vi "LVClass_WavefrontCorrectorSet ReadFile WavefrontCorrectorSetup.vi"(0 "WavefrontCorrectorSet in":refnum<class "WavefrontCorrectorSet.lvclass">, 11 "error in (no error)":errorcluster) -> (4 "WavefrontCorrectorSet out":refnum<class "WavefrontCorrectorSet.lvclass">, 15 "error out":errorcluster)   [LabVIEW 2020, in "WavefrontCorrectorSet.lvclass"]
uses:
  WavefrontCorrectorSet.lvclass
  WavefrontCorrectorSet.lvclass/WavefrontCorrectorSet.ctl
  CameraParametersSetup.ctl
  CameraParameters_Type.ctl
  File Exists - Scalar__ogtk.vi
  <vilib>/Utility/xml.llb/Read From XML File(string).vi
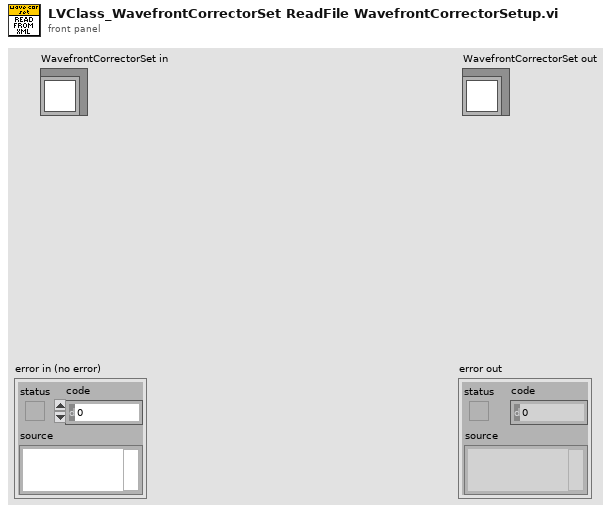
[diagram p1: front panel]
types:
  T1 = typedef "CameraParametersSetup.ctl" = cluster{"Name":string, "Type":T2, "Value":dbl, "BooleanValue":bool, "StringValue":string, "ConnectionParameter":bool}
  T2 = typedef "CameraParameters_Type.ctl" = enum16{"Integer", "Real", "String", "Boolean"}
  T3 = typedef "Wavefront Corrector states - ONE.ctl" = cluster{"Max":sgl, "Min":sgl, "Validity":enum16{"valid", "fixed", "invalid"}, "Fixed_Position":sgl}
  T4 = typedef "Wavefront Corrector states.ctl" = cluster{"Sleep after command apply_ms":i32, "Wavefront Corrector State":T3[], "WavefrontCorrectorOffsetState":sgl[]}
  T5 = typedef "ParameterID.ctl" = cluster{"Name":string, "ConnectionParameter?":bool, "Type":T2, "Authorization":T6, "OnFlyAuthorization":T7, "StringValue":string, "Value":dbl, "Min":dbl, "Max":dbl, "BooleanValue":bool, "StringParameterList":string[]}
  T6 = typedef "CameraParameters_Authorization.ctl" = enum16{"Disable", "Gettable", "Settable - Gettable"}
  T7 = typedef "CameraParameters_OnFlyAuthorization.ctl" = enum16{"None", "Gettable", "Settable", "Settable - Gettable"}
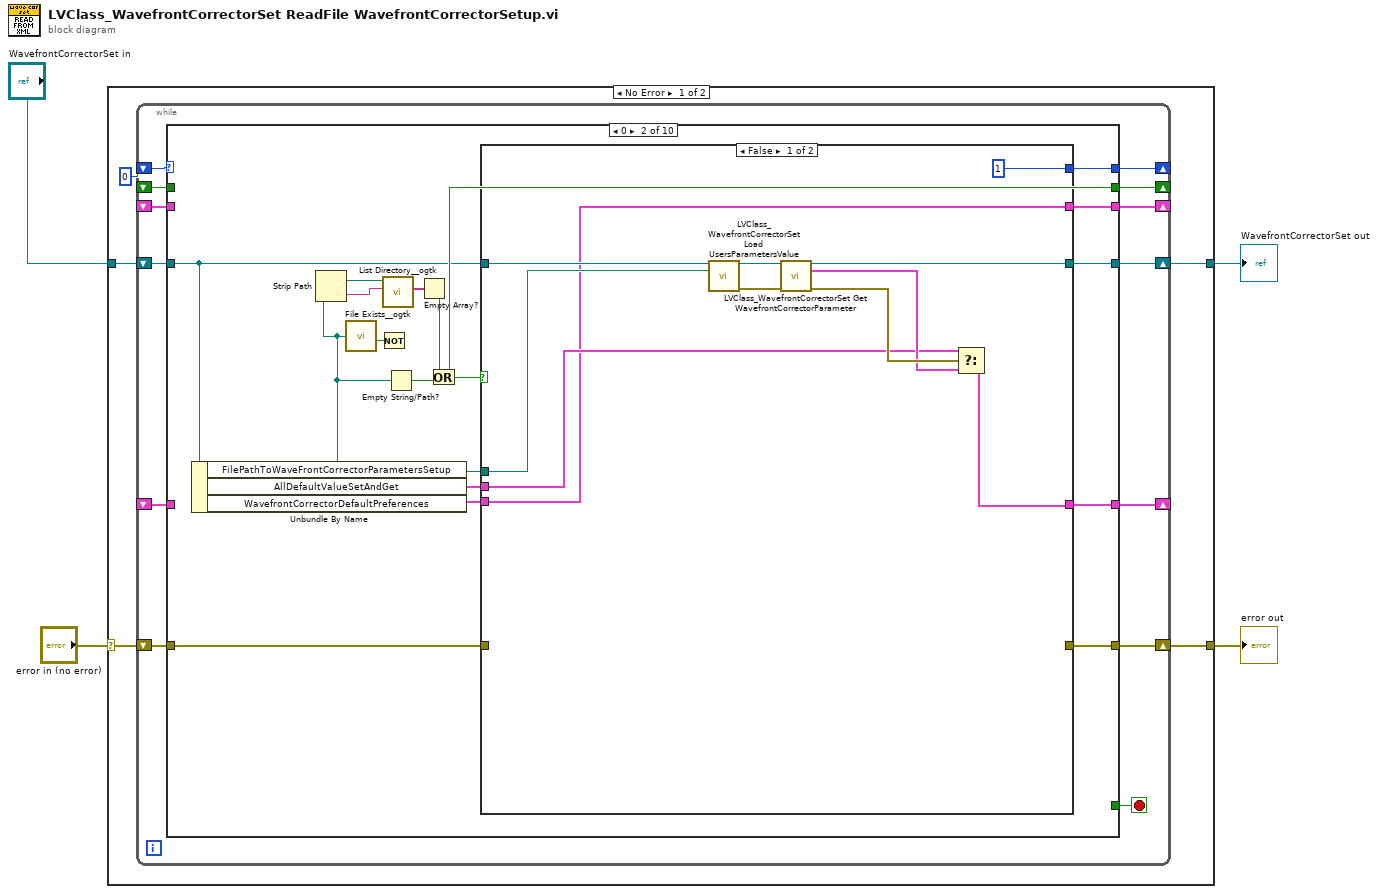
[diagram p0: block diagram]
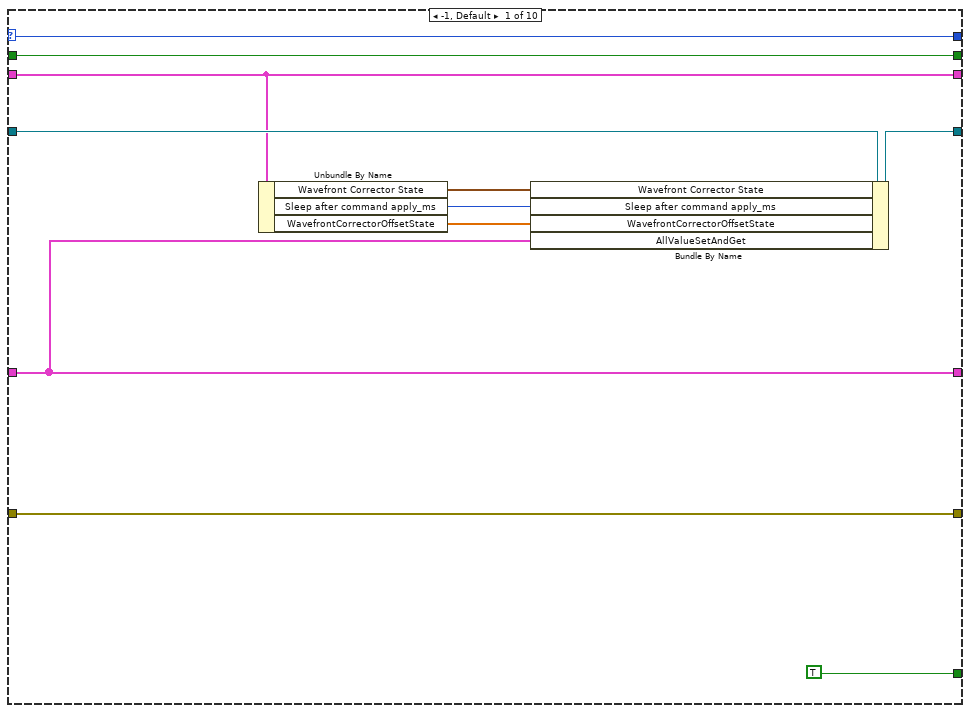
[diagram p2: hidden frame]
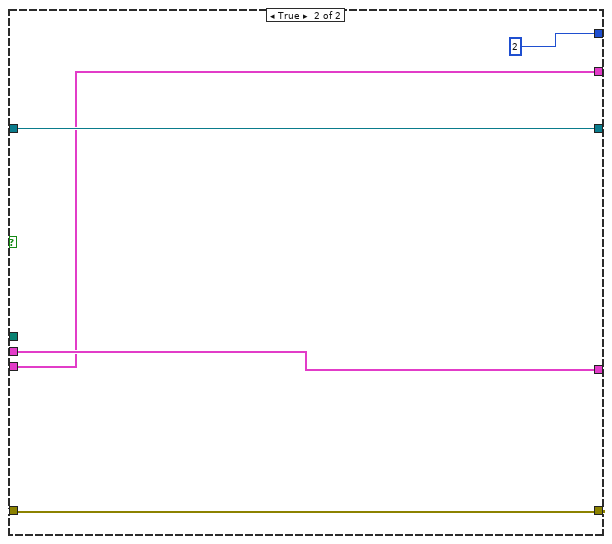
[diagram p3: hidden frame]
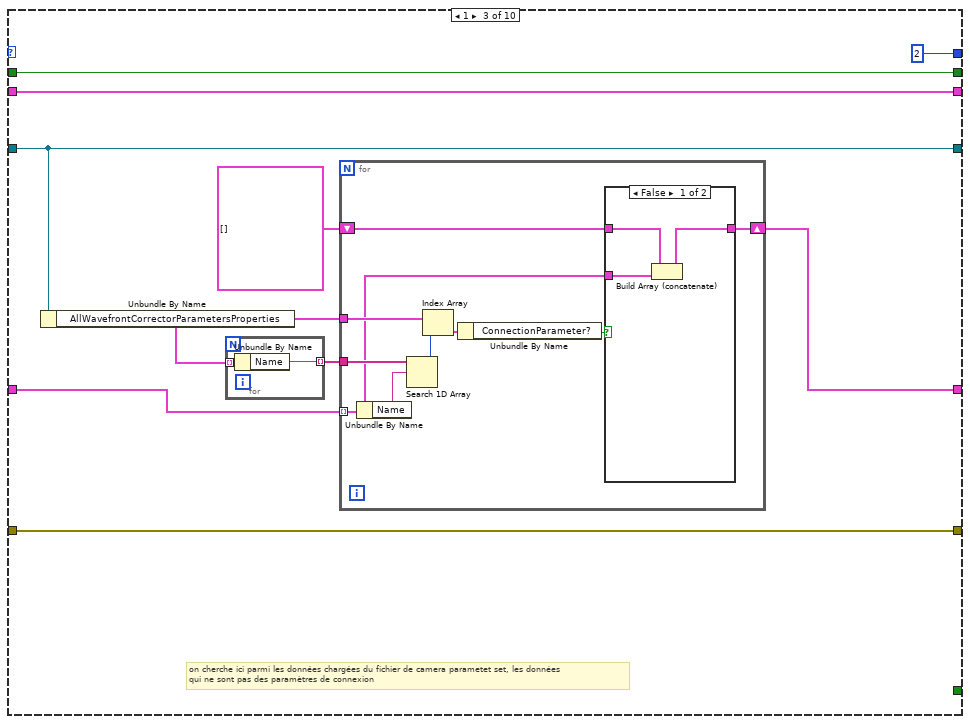
[diagram p4: hidden frame]
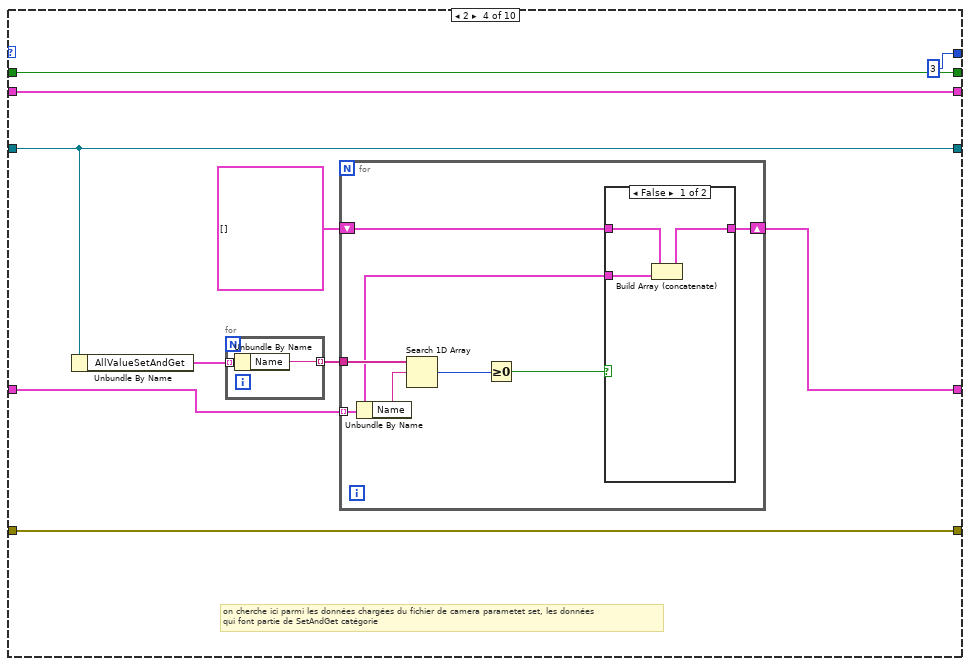
[diagram p6: hidden frame]
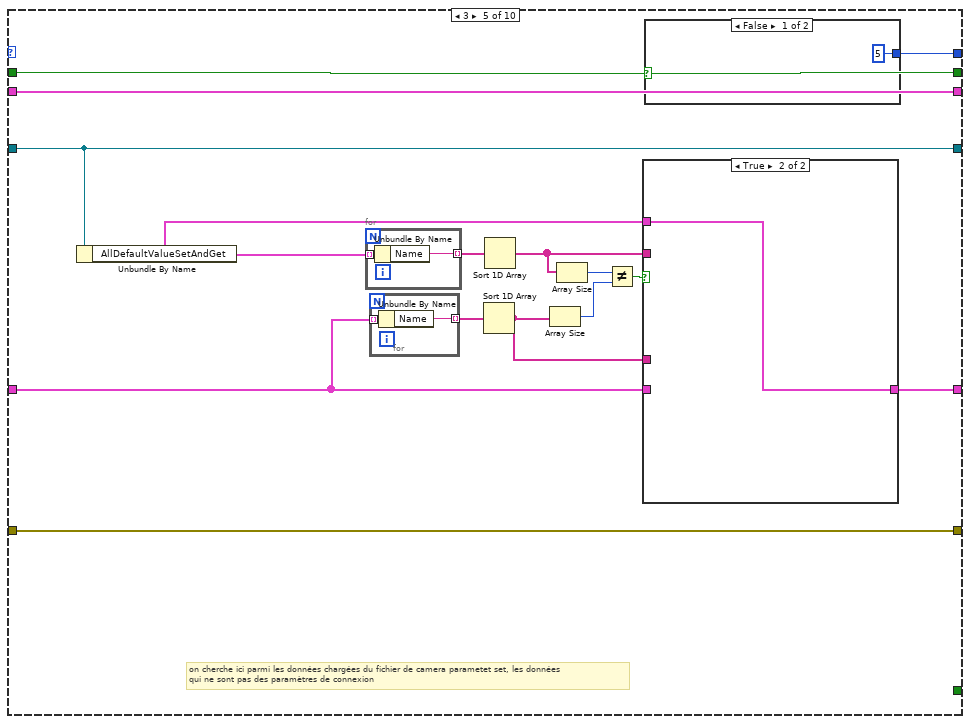
[diagram p8: hidden frame]
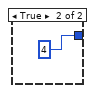
[diagram p9: hidden frame]
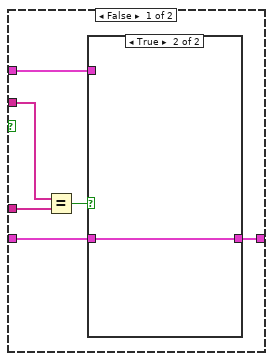
[diagram p10: hidden frame]
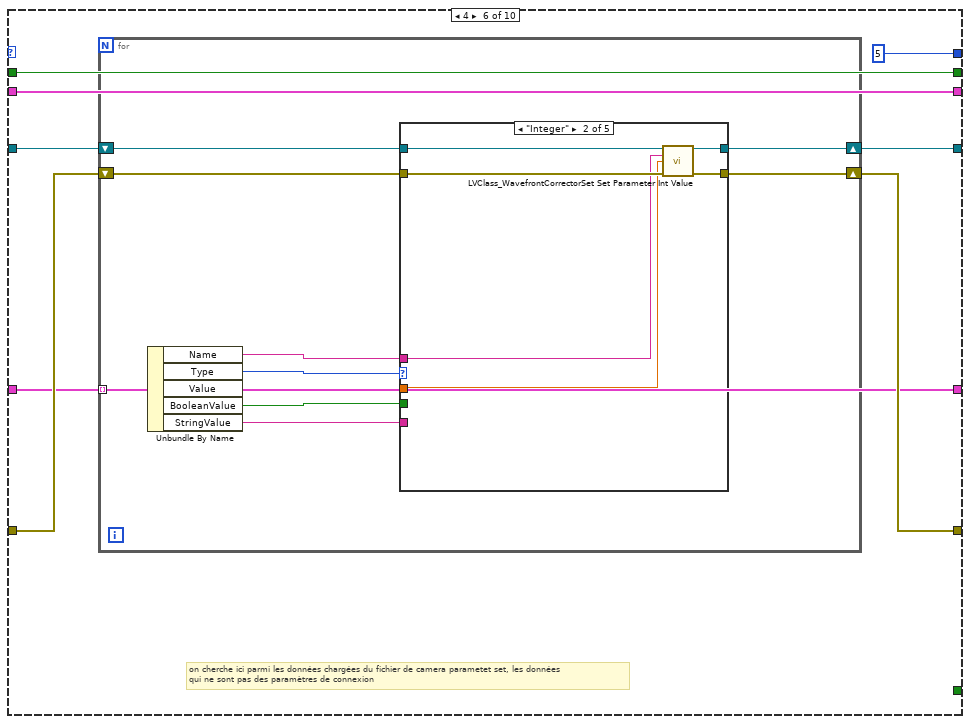
[diagram p12: hidden frame]
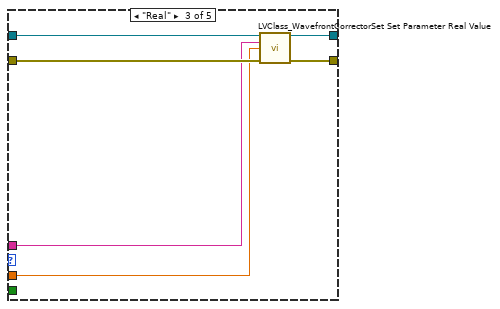
[diagram p14: hidden frame]
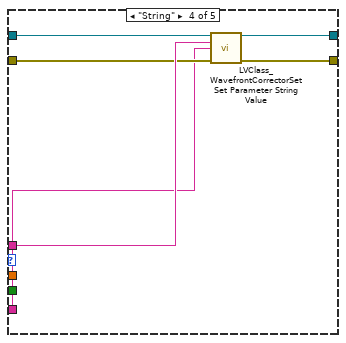
[diagram p15: hidden frame]
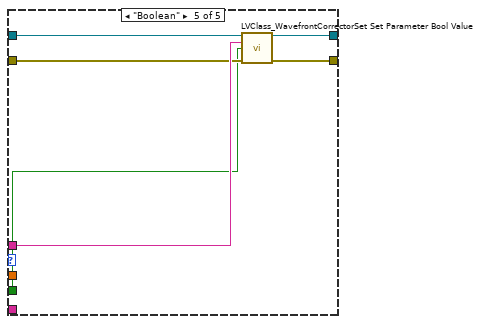
[diagram p16: hidden frame]
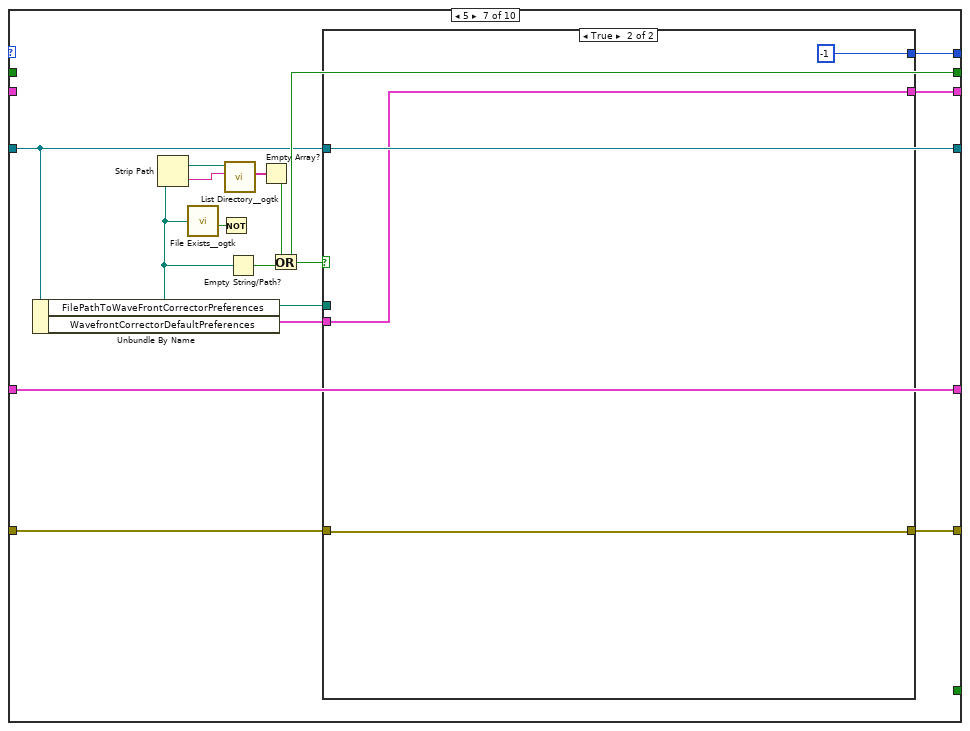
[diagram p17: hidden frame]
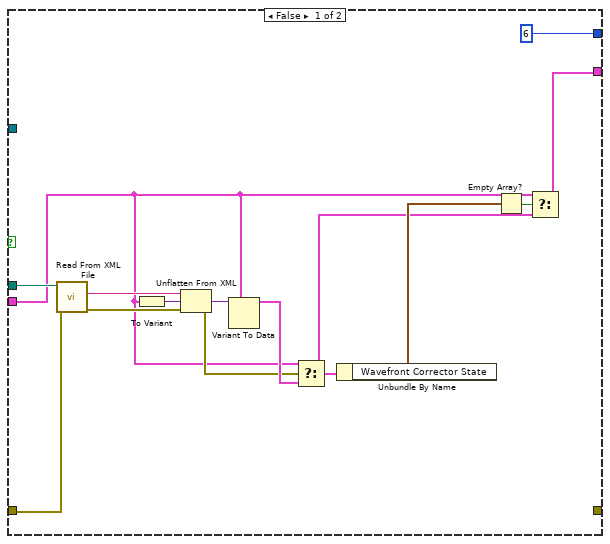
[diagram p18: hidden frame]
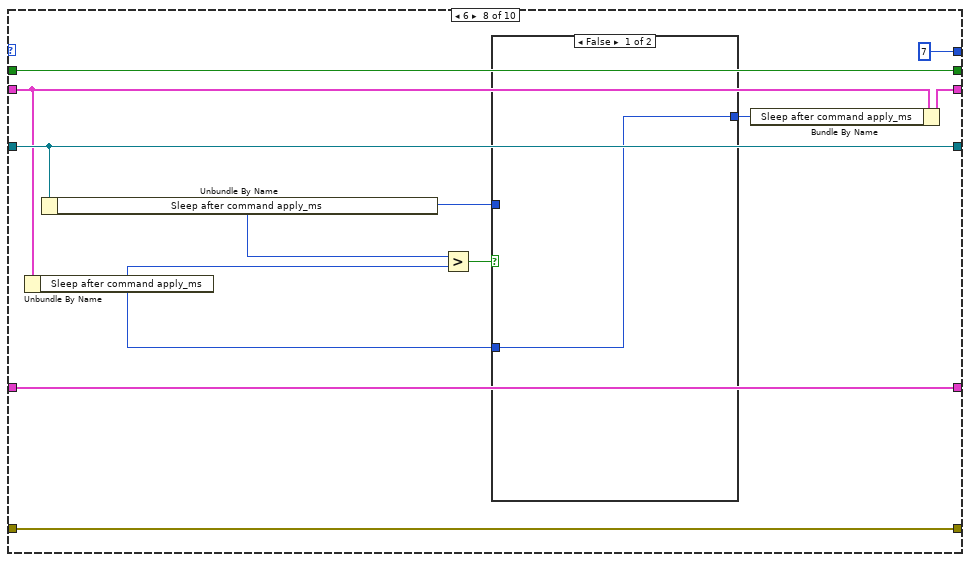
[diagram p19: hidden frame]
diagram:
  n1 = case shown="No Error" "error in (no error)" {
    selector: "error in (no error)" -> [w8 w265]
    tunnel: [w9 w265] -> w3
    tunnel: "WavefrontCorrectorSet in" -> [w6 w264]
    tunnel: [w5 w264] -> w1
    frame No Error {
      n2 = while {
        shift-right: [w20] -> _
        shift-left: _ -> [w16]
        shift-right: [w14] -> _
        shift-left: 0 -> [w18]
        shift-right: [w15] -> w5
        shift-left: w6 -> [w19]
        shift-right: [w22] -> w9
        shift-left: w8 -> [w21]
        shift-right: [w10] -> _
        shift-left: _ -> [w13]
        shift-right: [w11] -> _
        shift-left: _ -> [w12]
        stop <- w17 stop-if-true
        n3 = case shown="0" w18 {
          selector: w18 -> [w31 _ _ _ _ _ _ _ _ _]
          tunnel: [w32 w50 w75 w100 w124 w146 w203 w229 w241 w256] -> w22
          tunnel: w21 -> [w32 w49 w75 w100 w124 w147 w202 w229 w241 w256]
          tunnel: [w26 w48 w68 w93 w116 w150 w201 w221 w234 w249] -> w20
          tunnel: w19 -> [w30 w34 w71 w96 w129 w149 w189 w230 w245 w260]
          tunnel: [TRUE _ _ _ _ _ _ _ _ _] -> w17
          tunnel: w16 -> [w26 _ w68 w93 w116 w150 _ w222 w235 w250]
          tunnel: [w29 w37 w71 w96 w129 w148 w189 w230 w245 w260] -> w15
          tunnel: [w31 w46 2 3 w118 5 w200 7 8 -1] -> w14
          tunnel: [w27 w35 w69 w94 w119 w145 w190 w228 w238 w253] -> w10
          tunnel: w13 -> [w27 _ w70 w95 w117 w145 w190 w228 w238 w253]
          tunnel: w12 -> [w28 _ w67 w92 w115 w151 _ w224 w237 w252]
          tunnel: [w28 w36 w67 w92 w115 w151 w191 w224 w237 w252] -> w11
          frame -1, Default {
            n4 = Unbundle By Name(w26) -> ("Wavefront Corrector State"=w23:T3[], "Sleep after command apply_ms"=w24:i32, "WavefrontCorrectorOffsetState"=w25:sgl[])
            n5 = Bundle By Name(cluster=w30, "Wavefront Corrector State"=w23, "Sleep after command apply_ms"=w24, "WavefrontCorrectorOffsetState"=w25, "AllValueSetAndGet"=w27) -> (w29:refnum<class "WavefrontCorrectorSet.lvclass">)
          }
          frame 0 {
            n6 = Unbundle By Name(w34) -> ("FilePathToWaveFrontCorrectorParametersSetup"=w38:path, "AllDefaultValueSetAndGet"=w47:T1[], "WavefrontCorrectorDefaultPreferences"=w45:T4)
            n7 = Strip Path(path=w38) -> (stripped path=w41:path, name=w40:string)
            n8 = call-poly "File Exists__ogtk.vi"("file path"=w38) -> ("exists"=w39:bool)  [unwired: 6 in, 1 out]
            n9 = Not(x=w39) -> ()  [unwired: 1 out]
            n10 = call "List Directory__ogtk.vi"("pattern"=w40, "directory path"=w41) -> ("file names"=w42:string[])  [unwired: 2 in, 3 out]
            n11 = Empty String/Path?(string/path=w38) -> (empty?=w44:bool)
            n12 = Empty Array?(array=w42) -> (empty?=w43:bool)
            n13 = Or(x=w43, y=w44) -> (x .or. y?=w36:bool)
            n14 = case shown="False" w36 {
              tunnel: w38 -> [w58 _]
              tunnel: [_ w66] -> w50
              tunnel: w49 -> [_ w66]
              tunnel: [w51 w62] -> w48
              tunnel: w47 -> [w53 w63]
              tunnel: [1 2] -> w46
              tunnel: w45 -> [w51 w62]
              tunnel: w34 -> [w59 w64]
              tunnel: [w56 w64] -> w37
              tunnel: [w52 w63] -> w35
              frame False {
                n15 = call "LVClass_WavefrontCorrectorSet Load UsersParametersValue.vi"("WavefrontCorrectorSet in"=w59, "ParametersValue file path"=w58) -> ("WavefrontCorrectorSet out"=w57:refnum<class "WavefrontCorrectorSet.lvclass">, "error out"=w60:errorcluster)  [unwired: 12 in]
                n16 = call "LVClass_WavefrontCorrectorSet Get WavefrontCorrectorParameter.vi"("WavefrontCorrectorSet in"=w57, "error in (no error)"=w60) -> ("WavefrontCorrectorSet out"=w56:refnum<class "WavefrontCorrectorSet.lvclass">, "AllCurrentValueSetAndGet"=w54:T1[], "error out"=w55:errorcluster)  [unwired: 10 in, 1 out]
                n17 = Select(t=w53, s=w55, f=w54) -> (s? t:f=w52:T1[])
              }
              frame True {
              }
            }
          }
          frame 1 {
            # "on cherche ici parmi les données chargées du fichier de camera parametet set, les données \nqui ne sont pas des paramètres de connexion"
            n18 = Unbundle By Name(w71) -> ("AllWavefrontCorrectorParametersProperties"=w73:T5[])
            n19 = for {
              tunnel: w73 -> [w78] mode=indexing
              tunnel: [w77] -> w72 mode=indexing
              n20 = Unbundle By Name(w78) -> ("Name"=w77:string)
            }
            n21 = for {
              tunnel: w72 -> [w87]
              tunnel: w70 -> [w81] mode=indexing
              tunnel: w73 -> [w85]
              shift-right: [w82] -> w69
              shift-left: T1[] [] -> [w83]
              n22 = Unbundle By Name(w81) -> ("Name"=w86:string)
              n23 = Search 1D Array(1D array=w87, element=w86) -> (index of element=w84:i32)  [unwired: 1 in]
              n24 = Index Array(array=w85, index=w84) -> (element=w80:T5)
              n25 = Unbundle By Name(w80) -> ("ConnectionParameter?"=w79:bool)
              n26 = case shown="False" w79 {
                tunnel: w83 -> [w90 w91]
                tunnel: [w89 w91] -> w82
                tunnel: w81 -> [w88 _]
                frame False {
                  n27 = Build Array (concatenate)(w90, w88) -> (w89:T1[])
                }
                frame True {
                }
              }
            }
          }
          frame 2 {
            # "on cherche ici parmi les données chargées du fichier de camera parametet set, les données \nqui font partie de SetAndGet catégorie"
            n28 = Unbundle By Name(w96) -> ("AllValueSetAndGet"=w98:T1[])
            n29 = for {
              tunnel: w98 -> [w103] mode=indexing
              tunnel: [w102] -> w97 mode=indexing
              n30 = Unbundle By Name(w103) -> ("Name"=w102:string)
            }
            n31 = for {
              tunnel: w97 -> [w110]
              tunnel: w95 -> [w106] mode=indexing
              shift-right: [w107] -> w94
              shift-left: T1[] [] -> [w108]
              n32 = Unbundle By Name(w106) -> ("Name"=w109:string)
              n33 = Search 1D Array(1D array=w110, element=w109) -> (index of element=w105:i32)  [unwired: 1 in]
              n34 = Greater Or Equal To 0?(x=w105) -> (x >= 0?=w104:bool)
              n35 = case shown="False" w104 {
                tunnel: w108 -> [w113 w114]
                tunnel: [w112 w114] -> w107
                tunnel: w106 -> [w111 _]
                frame False {
                  n36 = Build Array (concatenate)(w113, w111) -> (w112:T1[])
                }
                frame True {
                }
              }
            }
          }
          frame 3 {
            # "on cherche ici parmi les données chargées du fichier de camera parametet set, les données \nqui ne sont pas des paramètres de connexion"
            n37 = Unbundle By Name(w129) -> ("AllDefaultValueSetAndGet"=w125:T1[])
            n38 = for {
              tunnel: w125 -> [w142] mode=indexing
              tunnel: [w141] -> w122 mode=indexing
              n39 = Unbundle By Name(w142) -> ("Name"=w141:string)
            }
            n40 = for {
              tunnel: w117 -> [w144] mode=indexing
              tunnel: [w143] -> w120 mode=indexing
              n41 = Unbundle By Name(w144) -> ("Name"=w143:string)
            }
            n42 = Sort 1D Array(array=w120) -> (sorted array=w121:string[])
            n43 = Sort 1D Array(array=w122) -> (sorted array=w123:string[])
            n44 = Array Size(array=w121) -> (size(s)=w127:i32)
            n45 = Array Size(array=w123) -> (size(s)=w128:i32)
            n46 = Not Equal?(x=w128, y=w127) -> (x != y?=w126:bool)
            n47 = case shown="True" w126 {
              tunnel: w125 -> [w132 w140]
              tunnel: [w134 w140] -> w119
              tunnel: w123 -> [w137 _]
              tunnel: w121 -> [w136 _]
              tunnel: w117 -> [w133 _]
              frame False {
                n48 = Equal?(x=w137, y=w136) -> (x = y?=w135:bool)
                n49 = case shown="True" w135 {
                  tunnel: [w138 w139] -> w134
                  tunnel: w133 -> [_ w139]
                  tunnel: w132 -> [w138 _]
                  frame False {
                  }
                  frame True {
                  }
                }
              }
              frame True {
              }
            }
            n50 = case shown="False" w115 {
              tunnel: [5 4] -> w118
              frame False {
              }
              frame True {
              }
            }
          }
          frame 4 {
            # "on cherche ici parmi les données chargées du fichier de camera parametet set, les données \nqui ne sont pas des paramètres de connexion"
            n51 = for {
              tunnel: w145 -> [w155] mode=indexing
              shift-right: [w156] -> w148
              shift-left: w149 -> [w157]
              shift-right: [w153] -> w146
              shift-left: w147 -> [w154]
              n52 = Unbundle By Name(w155) -> ("Name"=w158:string, "Type"=w162:T2, "Value"=w159:dbl, "BooleanValue"=w161:bool, "StringValue"=w160:string)
              n53 = case shown="\"Integer\"" w162 {
                tunnel: w158 -> [_ w165 w172 w181 w187]
                tunnel: w157 -> [w164 w170 w176 w182 w188]
                tunnel: [w164 w168 w174 w179 w185] -> w156
                tunnel: [w163 w167 w173 w178 w184] -> w153
                tunnel: w154 -> [w163 w169 w175 w180 w186]
                tunnel: w159 -> [_ w166 w171 _ _]
                tunnel: w161 -> [_ _ _ _ w183]
                tunnel: w160 -> [_ _ _ w177 _]
                frame Default {
                }
                frame "Integer" {
                  n54 = call "LVClass_WavefrontCorrectorSet Set Parameter Int Value.vi"("WavefrontCorrectorSet in"=w170, "parameter_name"=w165, "Value"=w166, "error in (no error)"=w169) -> ("WavefrontCorrectorSet out"=w168:refnum<class "WavefrontCorrectorSet.lvclass">, "error out"=w167:errorcluster)  [unwired: 10 in]
                }
                frame "Real" {
                  n55 = call "LVClass_WavefrontCorrectorSet Set Parameter Real Value.vi"("WavefrontCorrectorSet in"=w176, "parameter_name"=w172, "Value"=w171, "error in (no error)"=w175) -> ("WavefrontCorrectorSet out"=w174:refnum<class "WavefrontCorrectorSet.lvclass">, "error out"=w173:errorcluster)  [unwired: 10 in]
                }
                frame "String" {
                  n56 = call "LVClass_WavefrontCorrectorSet Set Parameter String Value.vi"("WavefrontCorrectorSet in"=w182, "parameter name"=w181, "Value"=w177, "error in (no error)"=w180) -> ("WavefrontCorrectorSet out"=w179:refnum<class "WavefrontCorrectorSet.lvclass">, "error out"=w178:errorcluster)  [unwired: 10 in]
                }
                frame "Boolean" {
                  n57 = call "LVClass_WavefrontCorrectorSet Set Parameter Bool Value.vi"("WavefrontCorrectorSet in"=w188, "parameter_name"=w187, "Value"=w183, "error in (no error)"=w186) -> ("WavefrontCorrectorSet out"=w185:refnum<class "WavefrontCorrectorSet.lvclass">, "error out"=w184:errorcluster)  [unwired: 10 in]
                }
              }
            }
          }
          frame 5 {
            n58 = Unbundle By Name(w189) -> ("FilePathToWaveFrontCorrectorPreferences"=w192:path, "WavefrontCorrectorDefaultPreferences"=w199:T4)
            n59 = Strip Path(path=w192) -> (stripped path=w195:path, name=w194:string)
            n60 = call-poly "File Exists__ogtk.vi"("file path"=w192) -> ("exists"=w193:bool)  [unwired: 6 in, 1 out]
            n61 = Not(x=w193) -> ()  [unwired: 1 out]
            n62 = call "List Directory__ogtk.vi"("pattern"=w194, "directory path"=w195) -> ("file names"=w196:string[])  [unwired: 2 in, 3 out]
            n63 = Empty String/Path?(string/path=w192) -> (empty?=w198:bool)
            n64 = Empty Array?(array=w196) -> (empty?=w197:bool)
            n65 = Or(x=w197, y=w198) -> (x .or. y?=w191:bool)
            n66 = case shown="True" w191 {
              tunnel: w192 -> [w206 _]
              tunnel: [_ w220] -> w203
              tunnel: w202 -> [w212 w220]
              tunnel: [w204 w218] -> w201
              tunnel: [6 -1] -> w200
              tunnel: w199 -> [w205 w218]
              tunnel: w189 -> [_ _]
              frame False {
                n67 = call-poly <vilib>:"Read From XML File.vi"("error in (no error)"=w212, "XML File Path"=w206) -> ("error out"=w208:errorcluster, "XML Elements"=w211:string)  [unwired: 7 in, 1 out]
                n68 = To Variant(anything=w205) -> (Variant=w210:variant)
                n69 = Unflatten From XML(xml string=w211, type=w210, error in (no error)=w208) -> (value=w209:variant, error out=w207:errorcluster)
                n70 = Variant To Data(type=w205, Variant=w209) -> (data=w213:T4)  [unwired: 1 in, 1 out]
                n71 = Select(t=w205, s=w207, f=w213) -> (s? t:f=w214:T4)
                n72 = Unbundle By Name(w214) -> ("Wavefront Corrector State"=w215:T3[])
                n73 = Empty Array?(array=w215) -> (empty?=w217:bool)
                n74 = Select(t=w205, s=w217, f=w214) -> (s? t:f=w204:T4)
              }
              frame True {
              }
            }
          }
          frame 6 {
            n75 = Unbundle By Name(w222) -> ("Sleep after command apply_ms"=w226:i32)
            n76 = Unbundle By Name(w230) -> ("Sleep after command apply_ms"=w227:i32)
            n77 = Greater?(x=w227, y=w226) -> (0:w225:bool)
            n78 = case shown="False" w225 {
              tunnel: w227 -> [_ w233]
              tunnel: w226 -> [w232 _]
              tunnel: [w232 w233] -> w223
              frame False {
              }
              frame True {
              }
            }
            n79 = Bundle By Name(cluster=w222, "Sleep after command apply_ms"=w223) -> (w221:T4)
          }
          frame 7 {
            n80 = Unbundle By Name(w235) -> ("Wavefront Corrector State"=w239:T3[])
            n81 = Unbundle By Name(w245) -> ("Wavefront Corrector State"=w240:T3[])
            n82 = Array Size(array=w240) -> (size(s)=w244:i32)
            n83 = Array Size(array=w239) -> (size(s)=w243:i32)
            n84 = Not Equal?(x=w244, y=w243) -> (x != y?=w242:bool)
            n85 = case shown="False" w242 {
              tunnel: w240 -> [_ w248]
              tunnel: [w247 w248] -> w236
              tunnel: w239 -> [w247 _]
              frame False {
              }
              frame True {
              }
            }
            n86 = Bundle By Name(cluster=w235, "Wavefront Corrector State"=w236) -> (w234:T4)
          }
          frame 8 {
            n87 = Unbundle By Name(w250) -> ("WavefrontCorrectorOffsetState"=w254:sgl[])
            n88 = Unbundle By Name(w260) -> ("WavefrontCorrectorOffsetState"=w255:sgl[])
            n89 = Array Size(array=w255) -> (size(s)=w259:i32)
            n90 = Array Size(array=w254) -> (size(s)=w258:i32)
            n91 = Not Equal?(x=w259, y=w258) -> (x != y?=w257:bool)
            n92 = case shown="False" w257 {
              tunnel: w255 -> [_ w263]
              tunnel: w254 -> [w262 _]
              tunnel: [w262 w263] -> w251
              frame False {
              }
              frame True {
              }
            }
            n93 = Bundle By Name(cluster=w250, "WavefrontCorrectorOffsetState"=w251) -> (w249:T4)
          }
        }
      }
    }
    frame Error {
    }
  }
  "error out" <- w3
  "WavefrontCorrectorSet out" <- w1
